vi "activateFilter.vi"(6 "Activate":bool, 8 "error in (no error)":errorcluster, 9 "Measurement Function":T1 items=["Current", "Charge", "Voltage", "Resistance"], 10 "Filter Type":T2, 11 "Electrometer in":refnum<class "Electrometer.lvclass">) -> (0 "error out":errorcluster, 3 "Electrometer out":refnum<class "Electrometer.lvclass">)   [LabVIEW 2016, in "Electrometer.lvclass"]
uses:
  Electrometer.lvclass
  filterType.ctl
  Modes.ctl
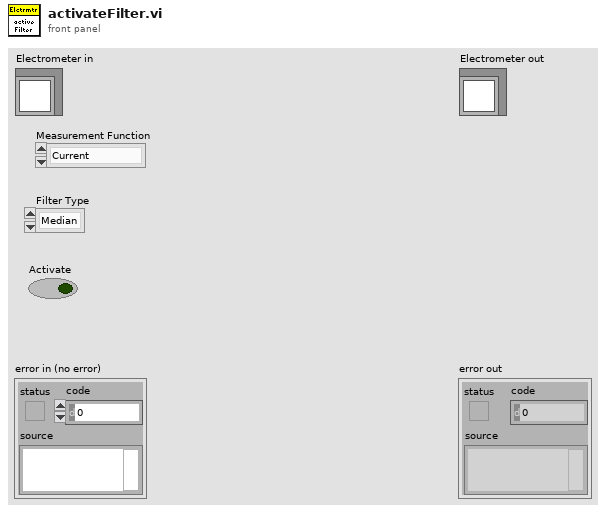
[diagram p1: front panel]
types:
  T1 = typedef "Electrometer.lvclass/Modes.ctl" = i32
  T2 = typedef "Electrometer.lvclass/filterType.ctl" = enum16{"Median", "Average"}
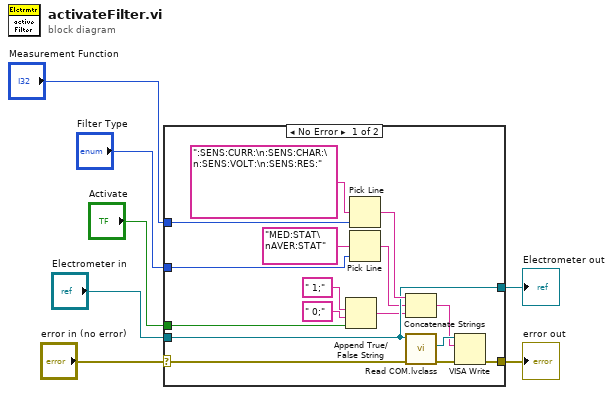
[diagram p0: block diagram]
diagram:
  n1 = case shown="No Error" "error in (no error)" {
    selector: "error in (no error)" -> [w16 w25]
    tunnel: [w15 w25] -> w6
    tunnel: [w18 w24] -> w4
    tunnel: "Electrometer in" -> [w18 w24]
    tunnel: "Activate" -> [w12 _]
    tunnel: "Measurement Function" -> [w17 _]
    tunnel: "Filter Type" -> [w13 _]
    frame No Error {
      n2 = Append True/False String(1:w12, 2:" 0;", 3:" 1;") -> (0:w10:string)  [unwired: 1 in]
      n3 = Pick Line(multi-line string=":SENS:CURR:\n:SENS:CHAR:\n:SENS:VOLT:\n:SENS:RES:", line index=w17) -> (output string=w20:string)  [unwired: 1 in]
      n4 = Pick Line(multi-line string="MED:STAT\nAVER:STAT", line index=w13) -> (output string=w11:string)  [unwired: 1 in]
      n5 = Concatenate Strings(w20, w11, w10) -> (w22:string)
      n6 = call "Read COM.lvclass.vi"("error in (no error)"=w16, "Electrometer in"=w18) -> ("error out"=w19:errorcluster, "VISA"=w23:refnum<visa-resource-name>)  [unwired: 7 in, 1 out]
      n7 = VISA Write(VISA resource name=w23, write buffer=w22, error in (no error)=w19) -> (error out=w15:errorcluster)  [unwired: 2 out]
    }
    frame Error {
    }
  }
  "error out" <- w6
  "Electrometer out" <- w4
